vi "写入数据地址处理.vi"(9 "输入2":u16[](array[numeric]), 10 "输入1":u16[](array[numeric])) -> (2 "完整帧":string)   [LabVIEW 2012]
panel:
  out "字符串":string
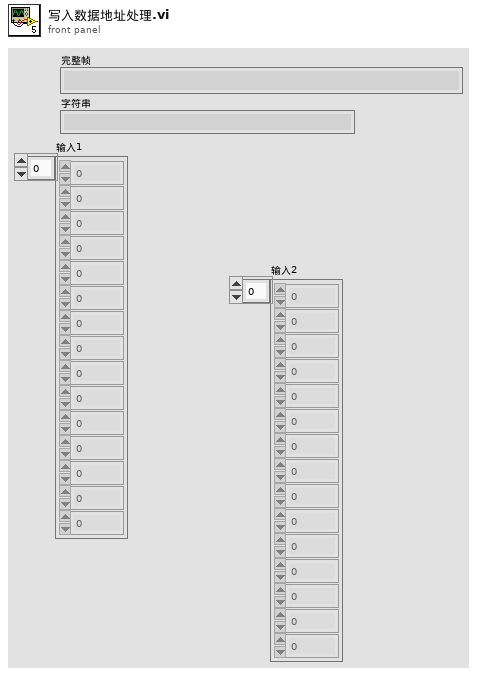
[diagram p1: front panel]
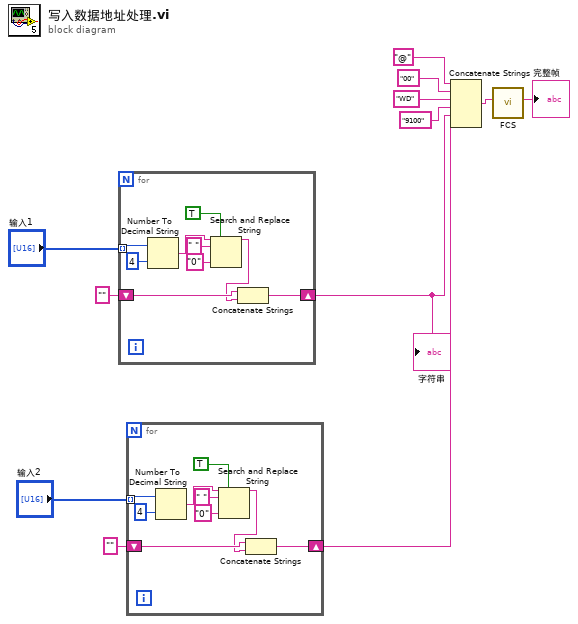
[diagram p0: block diagram]
diagram:
  n1 = for {
    tunnel: "输入1" -> [w21] mode=indexing
    shift-right: [w15] -> w5
    shift-left: "" -> [w14]
    n2 = Number To Decimal String(number=w21, width (-)=i16 4 ("宽度(-)")) -> (decimal integer string=w19:string)
    n3 = Search and Replace String(replace all?=TRUE ("替换全部？(F)"), input string=w19, search string=" " ("搜索字符串"), replace string="0" ("替换字符串(\"\")")) -> (result string=w13:string)  [unwired: 4 in, 3 out]
    n4 = Concatenate Strings(w14, w13) -> (w15:string)
  }
  "字符串" <- w5
  n5 = for {
    tunnel: "输入2" -> [w30] mode=indexing
    shift-right: [w24] -> w1
    shift-left: "" -> [w23]
    n6 = Number To Decimal String(number=w30, width (-)=i16 4 ("宽度(-)")) -> (decimal integer string=w28:string)
    n7 = Search and Replace String(replace all?=TRUE ("替换全部？(F)"), input string=w28, search string=" " ("搜索字符串"), replace string="0" ("替换字符串(\"\")")) -> (result string=w22:string)  [unwired: 4 in, 3 out]
    n8 = Concatenate Strings(w23, w22) -> (w24:string)
  }
  n9 = Concatenate Strings("@" ("字符串"), "00" ("字符串"), "WD" ("字符串"), "9100" ("字符串"), w5, w1) -> (w8:string)
  n10 = call "FCS.vi"("发送命令"=w8) -> ("完整帧"=→"完整帧":string)  [unwired: 9 in, 1 out]
